vi "MostrarRetardo.vi"(1 "Retardo":dbl) -> (0 "String Retardo":string)   [LabVIEW 2019]
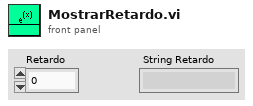
[diagram p1: front panel]
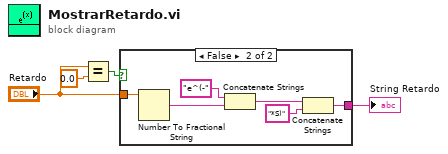
[diagram p0: block diagram]
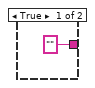
[diagram p2: hidden frame]
diagram:
  n1 = Equal?(x="Retardo", y=0.0) -> (x = y?=w2:bool)
  n2 = case shown="False" w2 {
    tunnel: "Retardo" -> [_ w11]
    tunnel: ["" w6] -> w1
    frame True {
    }
    frame False {
      n3 = Number To Fractional String(number=w11) -> (F-format string=w9:string)  [unwired: 3 in]
      n4 = Concatenate Strings("e^(-", w9) -> (w8:string)
      n5 = Concatenate Strings(w8, "*S)") -> (w6:string)
    }
  }
  "String Retardo" <- w1
